vi "8 Balls.vi"() -> ()   [LabVIEW 2019]
uses:
  Default8BallEnum.ctl
  JoysticksGlobal.vi
  MotorsGlobal.vi
  TurretMode.ctl
panel:
  in  "PID 8 Ball":T1(tab)
  in  "Distance1":dbl
  in  "DelayAnda1":i32=300
  in  "TimeLimit_Anda1":dbl
  in  "TimeLimit_AlinhaLL1":dbl
  in  "TimeLimit_Atira1":dbl
  in  "GainsCurvaDir1":T2={"proportional gain (Kc)"=1.0, "integral time (Ti, min)"=0.01, "derivative time (Td, min)"=0.0} {"derivative time (Td, min)" format="%.3f"; "integral time (Ti, min)" format="%.3f"; "proportional gain (Kc)" format="%.3f"}
  in  "RangeCurvaDir1":cluster{"output high":dbl, "output low":dbl}={"output high"=0.6, "output low"=-0.6} {"output low" format="%.2f"; "output high" format="%.2f"}
  in  "TimeLimit_CurvaDir1":dbl
  in  "Setpoint_CurvaDir1":dbl
  in  "Distance2":dbl
  in  "DelayAnda2":i32=300
  in  "TimeLimit_Anda2":dbl
  in  "GainsCurvaDir2":T2={"proportional gain (Kc)"=1.0, "integral time (Ti, min)"=0.01, "derivative time (Td, min)"=0.0} {"derivative time (Td, min)" format="%.3f"; "integral time (Ti, min)" format="%.3f"; "proportional gain (Kc)" format="%.3f"}
  in  "RangeCurvaDir2":cluster{"output high":dbl, "output low":dbl}={"output high"=0.6, "output low"=-0.6} {"output low" format="%.2f"; "output high" format="%.2f"}
  in  "TimeLimit_CurvaDir2":dbl
  in  "Setpoint_CurvaDir2":dbl
  in  "Distance3":dbl
  in  "DelayAnda3":i32=300
  in  "TimeLimit_Anda3":dbl
  in  "TimeLimit_AlinhaLL2":dbl
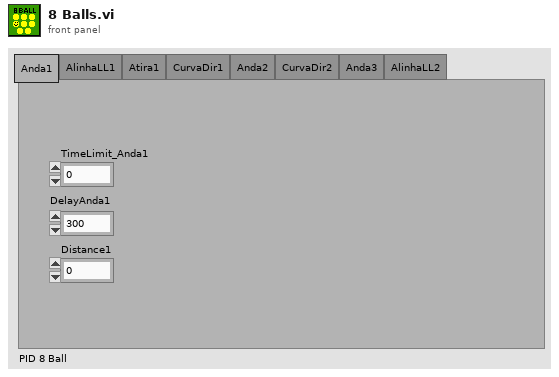
[diagram p1: front panel]
types:
  T1 = enum32{"Anda1", "AlinhaLL1", "Atira1", "CurvaDir1", "Anda2", "CurvaDir2", "Anda3", "AlinhaLL2"}
  T2 = cluster{"proportional gain (Kc)":dbl, "integral time (Ti, min)":dbl, "derivative time (Td, min)":dbl}
  T3 = typedef "TurretMode.ctl" = enum16{"Static", "Manual", "Automatic"}
  T4 = typedef "Default8BallEnum.ctl" = enum16{"Reset1", "Anda1", "AlinhaLL1", "Atira1", "CurvaDir1", "Reset2", "Anda2", "CurvaDir2", "Reset3", "Anda3", "AlinhaLL2", "Atira2"}
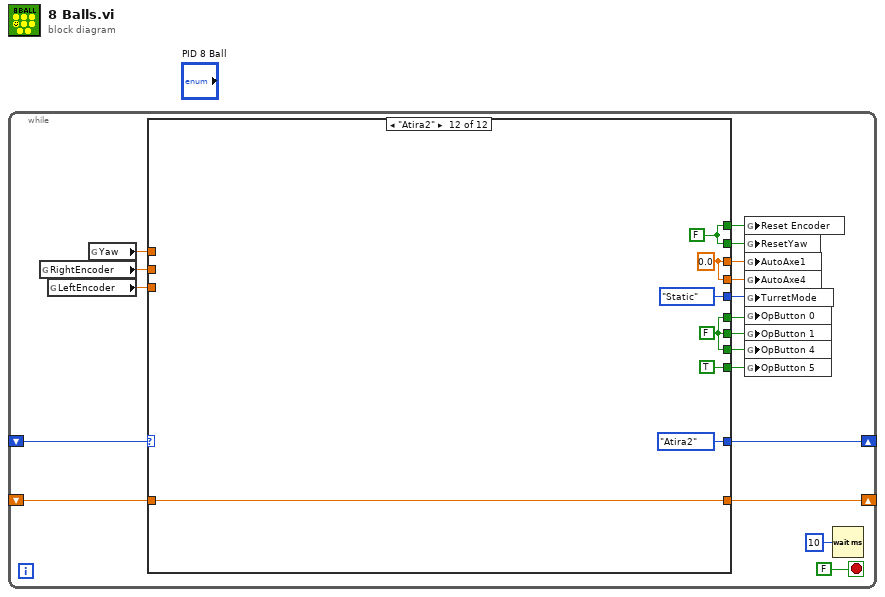
[diagram p0: block diagram]
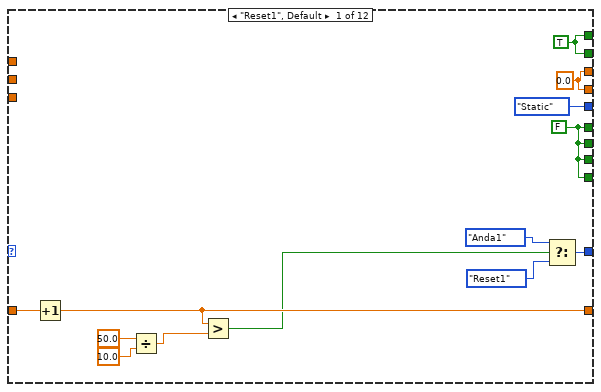
[diagram p2: hidden frame]
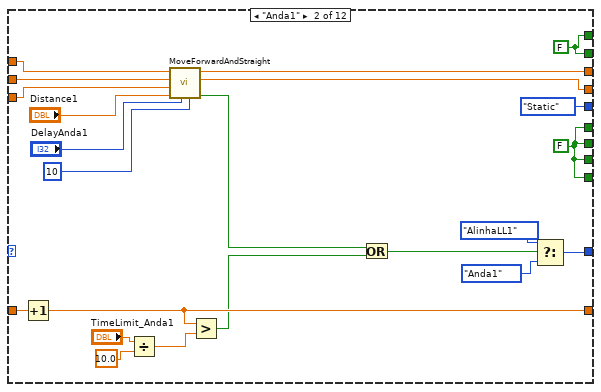
[diagram p3: hidden frame]
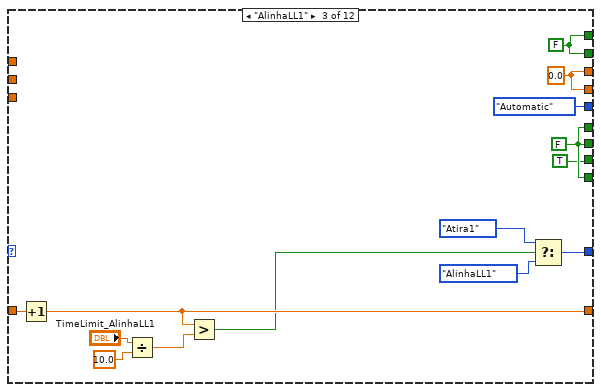
[diagram p4: hidden frame]
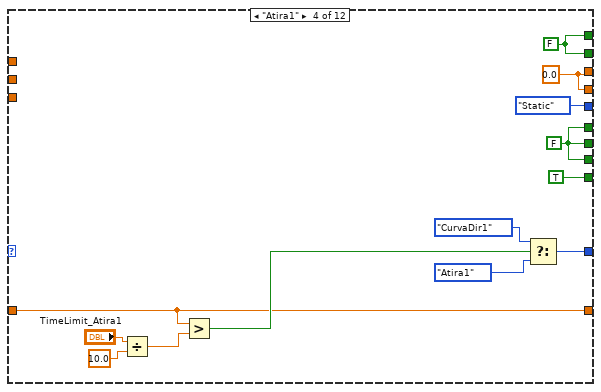
[diagram p5: hidden frame]
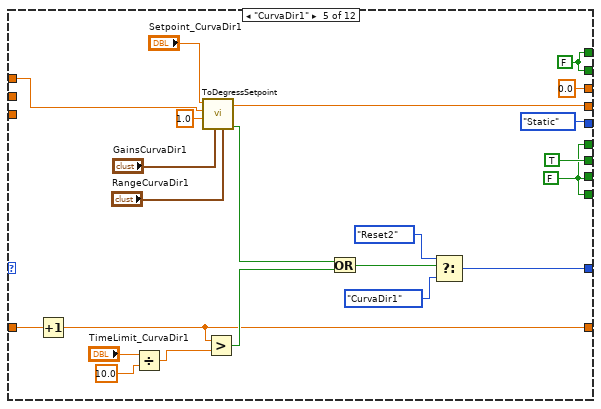
[diagram p6: hidden frame]
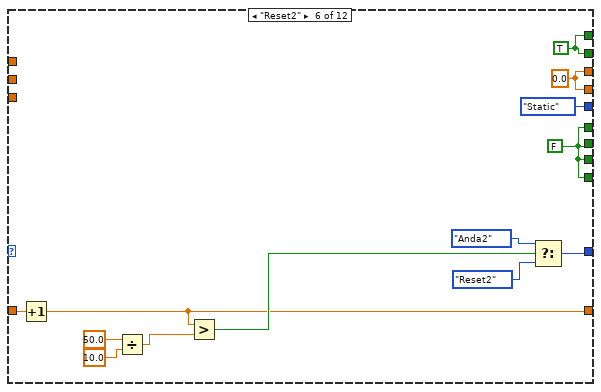
[diagram p7: hidden frame]
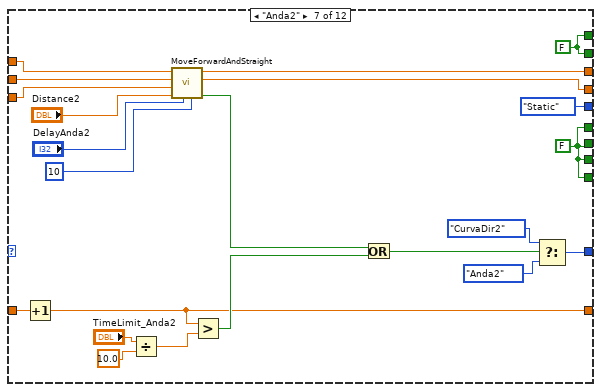
[diagram p8: hidden frame]
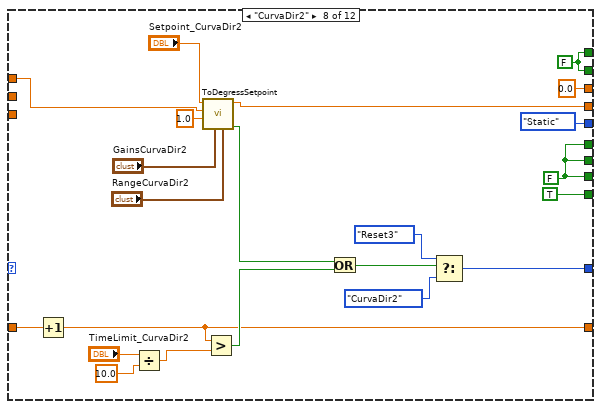
[diagram p9: hidden frame]
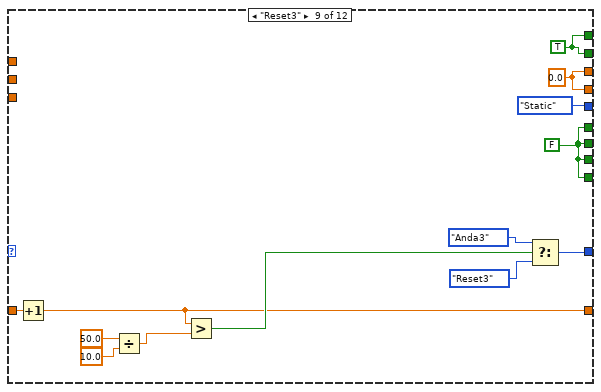
[diagram p10: hidden frame]
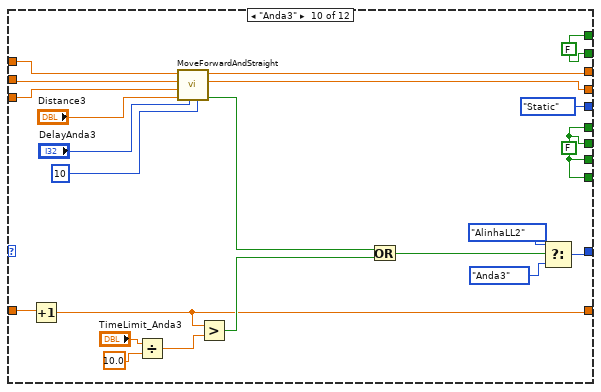
[diagram p11: hidden frame]
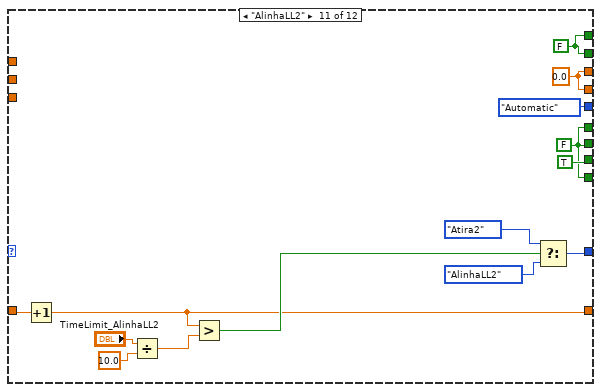
[diagram p12: hidden frame]
diagram:
  n1 = while {
    shift-right: [w15] -> _
    shift-left: _ -> [w16]
    shift-right: [w1] -> _
    shift-left: _ -> [w2]
    stop <- FALSE stop-if-true
    n2 = global read "MotorsGlobal.vi" "RightEncoder"() -> (w13:dbl)
    n3 = global read "MotorsGlobal.vi" "LeftEncoder"() -> (w12:dbl)
    n4 = global read "MotorsGlobal.vi" "Yaw"() -> (w14:dbl)
    n5 = case shown="\"Atira2\"" w16 {
      tunnel: [w31 w45 w57 w73 w92 w104 w124 w144 w164 w173 w199 Default8BallEnum."Atira2"] -> w15
      tunnel: w14 -> [_ w48 _ _ w89 _ w121 w147 _ w183 _ _]
      tunnel: w13 -> [_ w47 _ _ _ _ w120 _ _ w182 _ _]
      tunnel: w12 -> [_ w46 _ _ _ _ w119 _ _ w181 _ _]
      tunnel: [w28 w34 w63 w68 w87 w115 w122 w141 w166 w178 w200 w214] -> w11
      tunnel: [w28 w34 w63 w68 w87 w115 w122 w141 w166 w178 w200 w214] -> w10
      tunnel: [w27 w50 w64 w69 0.0 ("Trottle") w114 w117 0.0 ("Trottle") w162 w180 w195 w213] -> w9
      tunnel: [w27 w49 w64 w69 w86 w114 w118 w143 w162 w179 w195 w213] -> w8
      tunnel: [TurretMode."Static" ("TurretMode") TurretMode."Static" ("TurretMode") TurretMode."Automatic" ("TurretMode") TurretMode."Static" ("TurretMode") TurretMode."Static" ("TurretMode") TurretMode."Static" ("TurretMode") TurretMode."Static" ("TurretMode") TurretMode."Static" ("TurretMode") TurretMode."Static" ("TurretMode") TurretMode."Static" ("TurretMode") TurretMode."Automatic" ("TurretMode") TurretMode."Static" ("TurretMode")] -> w7
      tunnel: [w25 w33 w66 w71 w84 w112 w123 w140 w163 w177 w201 w212] -> w6
      tunnel: [w25 w33 w66 TRUE w84 w112 w123 TRUE w163 w177 w201 TRUE ("OpButton 0")] -> w5
      tunnel: [w25 w33 TRUE w71 w84 w112 w123 w140 w163 w177 TRUE w212] -> w4
      tunnel: [w25 w33 w66 w71 TRUE w112 w123 w140 w163 w177 w201 w212] -> w3
      tunnel: w2 -> [w22 w37 w59 w74 w82 w106 w126 w146 w160 w175 w198 w209]
      tunnel: [w21 w36 w58 w74 w81 w105 w125 w145 w165 w174 w197 w209] -> w1
      frame "Reset1", Default {
        w25 = FALSE ("OpButton 0")
        w27 = 0.0
        w28 = TRUE
        n6 = Increment(x=w22) -> (x+1=w21:dbl)
        n7 = Divide(x=50.0, y=10.0) -> (x/y=w23:dbl)
        n8 = Greater?(x=w21, y=w23) -> (0:w19:bool)
        n9 = Select(t=Default8BallEnum."Anda1", s=w19, f=Default8BallEnum."Reset1") -> (s? t:f=w31:T4)
      }
      frame "Anda1" {
        w34 = FALSE
        w33 = FALSE
        n10 = Increment(x=w37) -> (x+1=w36:dbl)
        n11 = Divide(x="TimeLimit_Anda1", y=10.0) -> (x/y=w39:dbl)
        n12 = call "MoveForwardAndStraight.vi"("Loop Timer"=10, "Time to stop"="DelayAnda1", "Distance"="Distance1", "Encoder Left"=w46, "Encoder Right"=w47, "Yaw"=w48) -> ("Finished distance"=w41:bool, "Direction"=w49:dbl, "Trottle"=w50:dbl)  [unwired: 2 in, 1 out]
        n13 = Greater?(x=w36, y=w39) -> (0:w35:bool)
        n14 = Or(x=w41, y=w35) -> (x .or. y?=w42:bool)
        n15 = Select(t=Default8BallEnum."AlinhaLL1", s=w42, f=Default8BallEnum."Anda1") -> (s? t:f=w45:T4)
      }
      frame "AlinhaLL1" {
        w63 = FALSE
        w64 = 0.0
        w66 = FALSE
        n16 = Increment(x=w59) -> (x+1=w58:dbl)
        n17 = Divide(x="TimeLimit_AlinhaLL1", y=10.0) -> (x/y=w61:dbl)
        n18 = Greater?(x=w58, y=w61) -> (0:w54:bool)
        n19 = Select(t=Default8BallEnum."Atira1", s=w54, f=Default8BallEnum."AlinhaLL1") -> (s? t:f=w57:T4)
      }
      frame "Atira1" {
        w68 = FALSE
        w69 = 0.0
        w71 = FALSE
        n20 = Divide(x="TimeLimit_Atira1", y=10.0) -> (x/y=w79:dbl)
        n21 = Greater?(x=w74, y=w79) -> (0:w75:bool)
        n22 = Select(t=Default8BallEnum."CurvaDir1", s=w75, f=Default8BallEnum."Atira1") -> (s? t:f=w73:T4)
      }
      frame "CurvaDir1" {
        w84 = FALSE
        w87 = FALSE
        n23 = Increment(x=w82) -> (x+1=w81:dbl)
        n24 = Divide(x="TimeLimit_CurvaDir1", y=10.0) -> (x/y=w100:dbl)
        n25 = call "ToDegressSetpoint.vi"("Range"="RangeCurvaDir1", "Gains"="GainsCurvaDir1", "Precision"=1.0, "Yaw"=w89, "Setpoint (degress)"="Setpoint_CurvaDir1") -> ("Finished?"=w93:bool, "Output"=w86:dbl)  [unwired: 5 in]
        n26 = Greater?(x=w81, y=w100) -> (0:w94:bool)
        n27 = Or(x=w93, y=w94) -> (x .or. y?=w95:bool)
        n28 = Select(t=Default8BallEnum."Reset2", s=w95, f=Default8BallEnum."CurvaDir1") -> (s? t:f=w92:T4)
      }
      frame "Reset2" {
        w112 = FALSE
        w114 = 0.0
        w115 = TRUE
        n29 = Increment(x=w106) -> (x+1=w105:dbl)
        n30 = Divide(x=50.0, y=10.0) -> (x/y=w109:dbl)
        n31 = Greater?(x=w105, y=w109) -> (0:w107:bool)
        n32 = Select(t=Default8BallEnum."Anda2", s=w107, f=Default8BallEnum."Reset2") -> (s? t:f=w104:T4)
      }
      frame "Anda2" {
        w122 = FALSE
        w123 = FALSE
        n33 = Increment(x=w126) -> (x+1=w125:dbl)
        n34 = Divide(x="TimeLimit_Anda2", y=10.0) -> (x/y=w129:dbl)
        n35 = call "MoveForwardAndStraight.vi"("Loop Timer"=10, "Time to stop"="DelayAnda2", "Distance"="Distance2", "Encoder Left"=w119, "Encoder Right"=w120, "Yaw"=w121) -> ("Finished distance"=w131:bool, "Direction"=w118:dbl, "Trottle"=w117:dbl)  [unwired: 2 in, 1 out]
        n36 = Greater?(x=w125, y=w129) -> (0:w127:bool)
        n37 = Or(x=w131, y=w127) -> (x .or. y?=w132:bool)
        n38 = Select(t=Default8BallEnum."CurvaDir2", s=w132, f=Default8BallEnum."Anda2") -> (s? t:f=w124:T4)
      }
      frame "CurvaDir2" {
        w140 = FALSE
        w141 = FALSE
        n39 = Increment(x=w146) -> (x+1=w145:dbl)
        n40 = Divide(x="TimeLimit_CurvaDir2", y=10.0) -> (x/y=w157:dbl)
        n41 = call "ToDegressSetpoint.vi"("Range"="RangeCurvaDir2", "Gains"="GainsCurvaDir2", "Precision"=1.0, "Yaw"=w147, "Setpoint (degress)"="Setpoint_CurvaDir2") -> ("Finished?"=w150:bool, "Output"=w143:dbl)  [unwired: 5 in]
        n42 = Greater?(x=w145, y=w157) -> (0:w151:bool)
        n43 = Or(x=w150, y=w151) -> (x .or. y?=w152:bool)
        n44 = Select(t=Default8BallEnum."Reset3", s=w152, f=Default8BallEnum."CurvaDir2") -> (s? t:f=w144:T4)
      }
      frame "Reset3" {
        w163 = FALSE
        w162 = 0.0
        w166 = TRUE
        n45 = Increment(x=w160) -> (x+1=w165:dbl)
        n46 = Divide(x=50.0, y=10.0) -> (x/y=w170:dbl)
        n47 = Greater?(x=w165, y=w170) -> (0:w168:bool)
        n48 = Select(t=Default8BallEnum."Anda3", s=w168, f=Default8BallEnum."Reset3") -> (s? t:f=w164:T4)
      }
      frame "Anda3" {
        w178 = FALSE
        w177 = FALSE
        n49 = Increment(x=w175) -> (x+1=w174:dbl)
        n50 = Divide(x="TimeLimit_Anda3", y=10.0) -> (x/y=w186:dbl)
        n51 = call "MoveForwardAndStraight.vi"("Loop Timer"=10, "Time to stop"="DelayAnda3", "Distance"="Distance3", "Encoder Left"=w181, "Encoder Right"=w182, "Yaw"=w183) -> ("Finished distance"=w188:bool, "Direction"=w179:dbl, "Trottle"=w180:dbl)  [unwired: 2 in, 1 out]
        n52 = Greater?(x=w174, y=w186) -> (0:w184:bool)
        n53 = Or(x=w188, y=w184) -> (x .or. y?=w189:bool)
        n54 = Select(t=Default8BallEnum."AlinhaLL2", s=w189, f=Default8BallEnum."Anda3") -> (s? t:f=w173:T4)
      }
      frame "AlinhaLL2" {
        w200 = FALSE
        w195 = 0.0
        w201 = FALSE
        n55 = Increment(x=w198) -> (x+1=w197:dbl)
        n56 = Divide(x="TimeLimit_AlinhaLL2", y=10.0) -> (x/y=w207:dbl)
        n57 = Greater?(x=w197, y=w207) -> (0:w203:bool)
        n58 = Select(t=Default8BallEnum."Atira2", s=w203, f=Default8BallEnum."AlinhaLL2") -> (s? t:f=w199:T4)
      }
      frame "Atira2" {
        w212 = FALSE ("OpButton 0")
        w213 = 0.0 ("Trottle")
        w214 = FALSE
      }
    }
    n59 = global write "MotorsGlobal.vi" "Reset Encoder"(w11) -> ()
    n60 = global write "MotorsGlobal.vi" "ResetYaw"(w10) -> ()
    n61 = global write "JoysticksGlobal.vi" "AutoAxe1"(w9) -> ()
    n62 = global write "JoysticksGlobal.vi" "AutoAxe4"(w8) -> ()
    n63 = global write "MotorsGlobal.vi" "TurretMode"(w7) -> ()
    n64 = global write "JoysticksGlobal.vi" "OpButton 0"(w6) -> ()
    n65 = global write "JoysticksGlobal.vi" "OpButton 1"(w3) -> ()
    n66 = global write "JoysticksGlobal.vi" "OpButton 4"(w4) -> ()
    n67 = global write "JoysticksGlobal.vi" "OpButton 5"(w5) -> ()
    n68 = Wait (ms)(milliseconds to wait=u32 10) -> ()  [unwired: 1 out]
  }
